vi "Simple Tank Simulation using Button.vi"() -> ()   [LabVIEW 2021]
panel:
  in  "stop":bool
  out "Tank":dbl(slide) scale=0.0..100.0
  in  "OK Button":bool
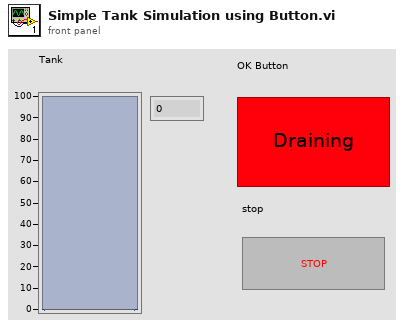
[diagram p1: front panel]
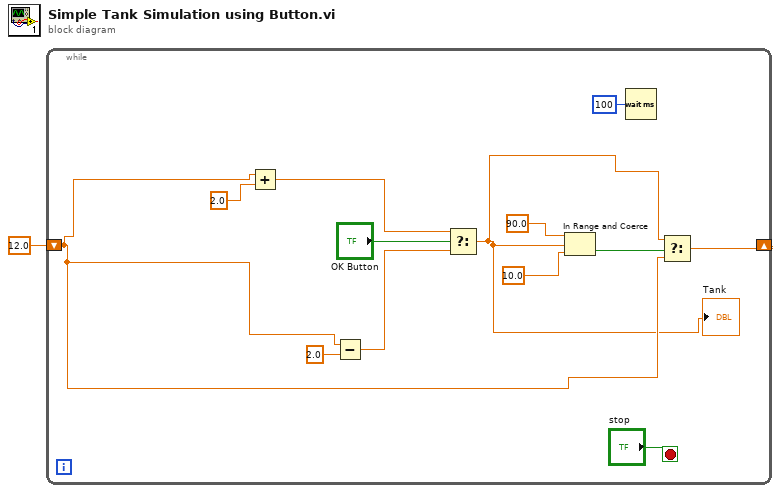
[diagram p0: block diagram]
diagram:
  n1 = while {
    shift-right: [w8] -> _
    shift-left: 12.0 -> [w3]
    stop <- "stop" stop-if-true
    n2 = Add(x=w3, y=2.0) -> (x+y=w13:dbl)
    n3 = Subtract(x=w3, y=2.0) -> (x-y=w12:dbl)
    n4 = Select(t=w13, s="OK Button", f=w12) -> (s? t:f=w2:dbl)
    "Tank" <- w2
    n5 = In Range and Coerce(upper limit=90.0, x=w2, lower limit=10.0) -> (In Range?=w7:bool)  [unwired: 1 out]
    n6 = Wait (ms)(milliseconds to wait=u32 100) -> ()  [unwired: 1 out]
    n7 = Select(t=w2, s=w7, f=w3) -> (s? t:f=w8:dbl)
  }
